vi "Write Cal Tone Site.vi"(8 "error in (no error)":errorcluster, 10 "Cal Tone Site":i32, 11 "SA Path in":refnum<class "SA Path.lvclass">) -> (0 "error out":errorcluster, 3 "SA Path out":refnum<class "SA Path.lvclass">)   [LabVIEW 2023, in "RFFixtureCharact.Public.lvlib" / "SA Path.lvclass"]
uses:
  SA Path.lvclass
  SA Path.lvclass/SA Path.ctl
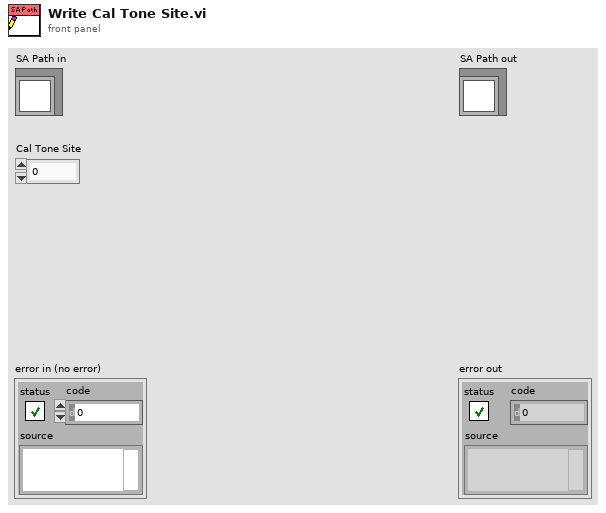
[diagram p1: front panel]
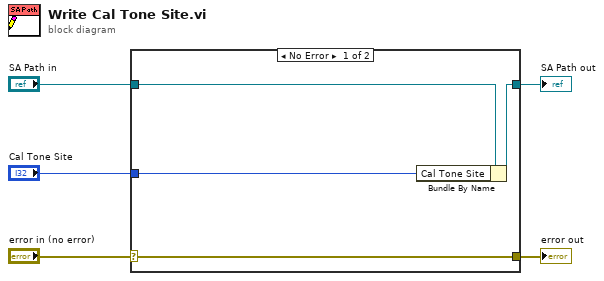
[diagram p0: block diagram]
diagram:
  n1 = case shown="No Error" "error in (no error)" {
    selector: "error in (no error)" -> [w9 w10]
    tunnel: [w9 w10] -> w4
    tunnel: [w7 w11] -> w2
    tunnel: "SA Path in" -> [w8 w11]
    tunnel: "Cal Tone Site" -> [w6 _]
    frame No Error {
      n2 = Bundle By Name(cluster=w8, "Cal Tone Site"=w6) -> (w7:refnum<class "SA Path.lvclass">)
    }
    frame Error {
    }
  }
  "error out" <- w4
  "SA Path out" <- w2
